vi "Set_Hi-Tec_server.vi"(4 "Client Name":string, 6 "Density Ratio":string, 7 "Strength (% by volume)":dbl min=0.0 max=5.0 format="%.3f", 8 "Stack flowrate (l/min)":dbl format="%.2f", 9 "Mode":enum16{"Control Hi-Tec", "Check Hi-Tec Demands"}(ring)) -> (0 "Flowrates (kg/min)":dbl[](array[numeric]) format="%.2f", 1 "Comment":string)   [LabVIEW 2010]
uses:
  ADAM Client/Sub VIs/ADAM Controls/Update_scan_value.ctl
  ADAM Client/Sub VIs/ADAM Controls/Ch_description_ADAM.ctl
  ADAM Client/Sub VIs/ADAM Controls/Module_type_ADAM.ctl
  ADAM Client/Sub VIs/ADAM Controls/Function_ADAM.ctl
  ADAM Client/Sub VIs/ADAM Controls/Channel_State.ctl
  ADAM Client/Sub VIs/ADAM Controls/Calib_type_ADAM.ctl
  ADAM Client/Sub VIs/ADAM Controls/Address.ctl
  Anemometry/Anemometry Sub Vis/Globals/Gas_management_global.vi
panel:
  # "-Carrier 1 only\n-Carrier 2 only\n-Enter Ratio"
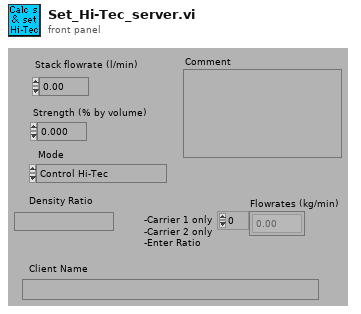
[diagram p1: front panel]
types:
  T1 = enum16{"Append to Global", "Read Global then Clear"}
  T2 = typedef "Ch_description_ADAM.ctl" = cluster{"Ch Name":string, "Type":T3, "Function":T4, "Ch State":T5, "Calibration type":T6, "A":dbl, "B":dbl, "C":dbl, "D":dbl, "Comments":string, "Address":T7, "String":string, "Duty":u16}
  T3 = typedef "Module_type_ADAM.ctl" = enum16{"4011", "4012", "4013", "4014", "4016", "4017", "4018", "4021", "4050", "4052", "4053", "4060", "4080", "5000", "5017", "5018", "5024", "5051", "5056", "5060", "6060", "Tracker", "WEST", "GILL", "JEM", "VICI", "Vaisala", "DRUCK", "Run VI Named:", "IR2100", "PPT", "Comparator", "VIRTUAL", "Hold Value", "Read A", "Read Ch", "Coded", "Client Info", "Web Client", "X10", "Test"}
  T4 = typedef "Function_ADAM.ctl" = enum16{"Analogue Input", "Digital Input", "Event counter", "Event rate", "Analogue Output", "Digital Output", "Relay Output"}
  T5 = typedef "Channel_State.ctl" = enum16{"On", "Off", "Always On", "Always Off"}
  T6 = typedef "Calib_type_ADAM.ctl" = enum16{"Raw", "Bx + A", "Cx^2 + Bx + A", "Dx^3 + Cx^2 + Bx + A", "In Band", "Hi-Tec Q", "Hi-Tec M_dot", "Text"}
  T7 = typedef "Address.ctl" = cluster{"Main":i32, "Ch.":i32, "Sub":i32, "Port Name":string}
  T8 = typedef "Update_scan_value.ctl" = cluster{"Channel Name":string, "New Value":dbl}
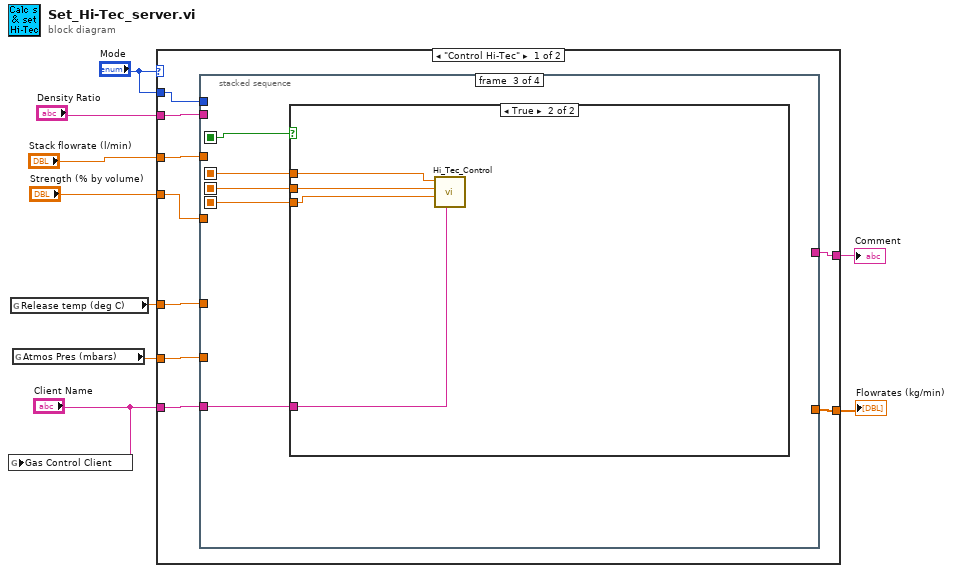
[diagram p0: block diagram]
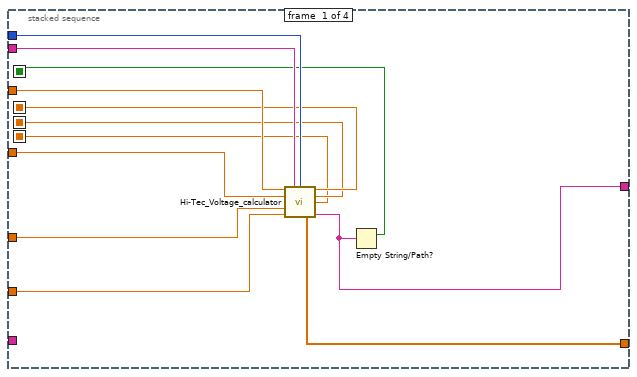
[diagram p2: hidden frame]
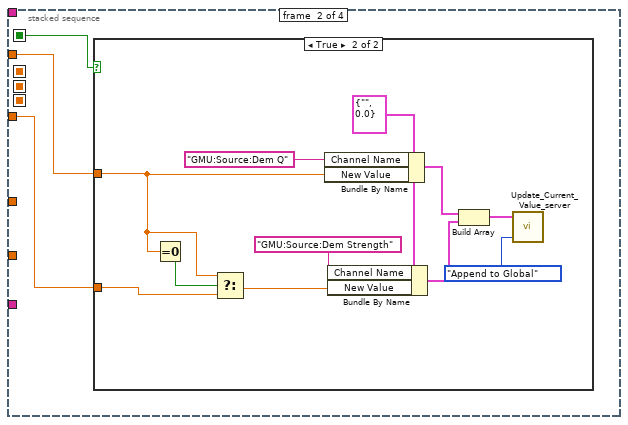
[diagram p3: hidden frame]
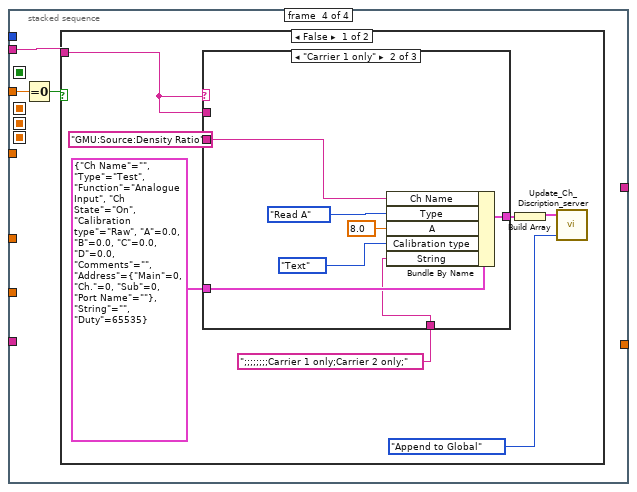
[diagram p6: hidden frame]
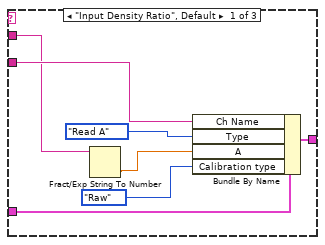
[diagram p7: hidden frame]
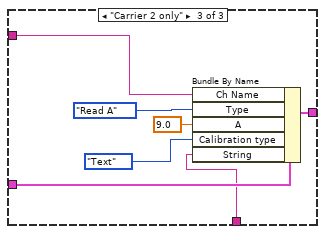
[diagram p8: hidden frame]
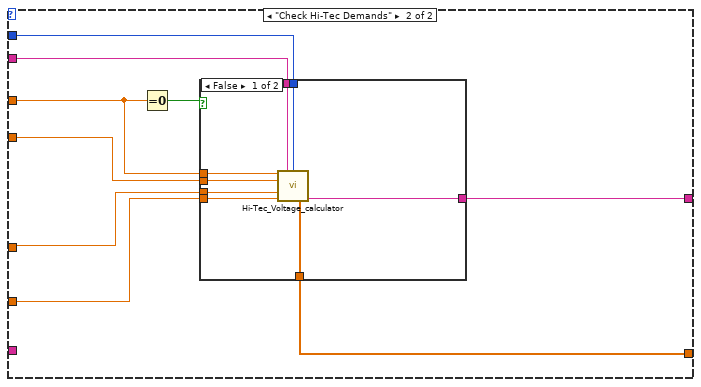
[diagram p10: hidden frame]
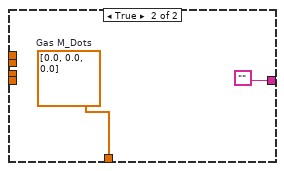
[diagram p11: hidden frame]
diagram:
  n1 = global write "Gas_management_global.vi" "Gas Control Client"("Client Name") -> ()
  n2 = global read "Gas_management_global.vi" "Release temp (deg C)"() -> (w5:dbl)
  n3 = global read "Gas_management_global.vi" "Atmos Pres (mbars)"() -> (w7:dbl)
  n4 = case shown="\"Control Hi-Tec\"" "Mode" {
    tunnel: "Density Ratio" -> [w18 w90]
    tunnel: "Strength (% by volume)" -> [w17 w93]
    tunnel: "Stack flowrate (l/min)" -> [w16 w88]
    tunnel: w5 -> [w15 w92]
    tunnel: w7 -> [w14 w91]
    tunnel: [w13 w89] -> w6
    tunnel: [w12 w86] -> w3
    tunnel: "Mode" -> [w11 w85]
    tunnel: "Client Name" -> [w10 _]
    frame "Control Hi-Tec" {
      n5 = stacked-sequence {
        seq-local: [w22 _ _ _] -> [_ w31 w45 _]
        seq-local: [w21 _ _ _] -> [_ _ w49 _]
        seq-local: [w20 _ _ _] -> [_ _ w48 _]
        seq-local: [w19 _ _ _] -> [_ _ w47 _]
        tunnel: w18 -> [w28 _ _ w56]
        tunnel: w17 -> [w27 w32 _ _]
        tunnel: w16 -> [w26 w33 _ w55]
        tunnel: w15 -> [w30 _ _ _]
        tunnel: w14 -> [w29 _ _ _]
        tunnel: [w23 _ _ _] -> w13
        tunnel: [w25 _ _ _] -> w12
        tunnel: w11 -> [w24 _ _ _]
        tunnel: w10 -> [_ _ w46 _]
        frame #0 {
          n6 = call "Hi-Tec_Voltage_calculator.vi"("Stack Flowrate (l/min)"=w26, "Density Ratio"=w28, "Mode"=w24, "Strength (% by volume)"=w27, "Release temp (deg C)"=w30, "Atmos Pres (mbars)"=w29) -> ("Carrier 1 Voltage"=w21:dbl, "Carrier 2 Voltage"=w20:dbl, "Trace Voltage"=w19:dbl, "Flowrates (kg/min)"=w25:dbl[], "Error Comments"=w23:string)  [unwired: 2 in, 3 out]
          n7 = Empty String/Path?(string/path=w23) -> (empty?=w22:bool)
        }
        frame #1 {
          n8 = case shown="True" w31 {
            tunnel: w33 -> [_ w44]
            tunnel: w32 -> [_ w43]
            frame False {
            }
            frame True {
              w38 = T8 {"Channel Name"="", "New Value"=0.0} ("Update Scan Value Cluster")
              n9 = Equal To 0?(x=w44) -> (x = 0?=w35:bool)
              n10 = Select(t=w44, s=w35, f=w43) -> (s? t:f=w34:dbl)
              n11 = Bundle By Name(cluster=w38, "Channel Name"="GMU:Source:Dem Q", "New Value"=w44) -> (w41:T8)
              n12 = Bundle By Name(cluster=w38, "Channel Name"="GMU:Source:Dem Strength", "New Value"=w34) -> (w42:T8)
              n13 = Build Array(w41, w42) -> (w37:T8[])
              n14 = call "Update_Current_Value_server.vi"("Mode"=T1."Append to Global", "Update array in"=w37) -> ()  [unwired: 1 in, 1 out]
            }
          }
        }
        frame #2 {
          n15 = case shown="True" w45 {
            tunnel: w49 -> [_ w53]
            tunnel: w48 -> [_ w52]
            tunnel: w47 -> [_ w51]
            tunnel: w46 -> [_ w50]
            frame False {
            }
            frame True {
              n16 = call "Hi_Tec_Control.vi"("Carrier 1 Voltage"=w53, "Carrier 2 Voltage"=w52, "Trace Voltage"=w51, "Client Name"=w50) -> ()  [unwired: 3 out]
            }
          }
        }
        frame #3 {
          n17 = Equal To 0?(x=w55) -> (x = 0?=w54:bool)
          n18 = case shown="False" w54 {
            tunnel: w56 -> [w58 _]
            frame False {
              n19 = case shown="\"Carrier 1 only\"" w58 {
                tunnel: T2 {"Ch Name"="", "Type"=enum."Test", "Function"=enum."Analogue Input", "Ch State"=enum."On", "Calibration type"=enum."Raw", "A"=0.0, "B"=0.0, "C"=0.0, "D"=0.0, "Comments"="", "Address"={"Main"=0, "Ch."=0, "Sub"=0, "Port Name"=""}, "String"="", "Duty"=65535} ("Ch Discription") -> [w70 w77 w84]
                tunnel: "GMU:Source:Density Ratio" -> [w69 w76 w83]
                tunnel: [w66 w72 w79] -> w61
                tunnel: w58 -> [w64 _ _]
                tunnel: ";;;;;;;;Carrier 1 only;Carrier 2 only;" -> [_ w71 w78]
                frame "Input Density Ratio", Default {
                  n20 = Fract/Exp String To Number(string=w64) -> (number=w65:dbl)  [unwired: 4 out]
                  n21 = Bundle By Name(cluster=w70, "Ch Name"=w69, "Type"=Module_type_ADAM."Read A", "A"=w65, "Calibration type"=Calib_type_ADAM."Raw") -> (w66:T2)
                }
                frame "Carrier 1 only" {
                  n22 = Bundle By Name(cluster=w77, "Ch Name"=w76, "Type"=Module_type_ADAM."Read A", "A"=8.0 ("Bundle Element"), "Calibration type"=Calib_type_ADAM."Text", "String"=w71) -> (w72:T2)
                }
                frame "Carrier 2 only" {
                  n23 = Bundle By Name(cluster=w84, "Ch Name"=w83, "Type"=Module_type_ADAM."Read A", "A"=9.0 ("Bundle Element"), "Calibration type"=Calib_type_ADAM."Text", "String"=w78) -> (w79:T2)
                }
              }
              n24 = Build Array(w61) -> (w60:T2[])
              n25 = call "Update_Ch_Discription_server.vi"("Mode"=T1."Append to Global", "Channels to update In"=w60) -> ()  [unwired: 1 in, 1 out]
            }
            frame True {
            }
          }
        }
      }
    }
    frame "Check Hi-Tec Demands" {
      n26 = Equal To 0?(x=w88) -> (x = 0?=w87:bool)
      n27 = case shown="False" w87 {
        tunnel: w93 -> [w101 _]
        tunnel: w92 -> [w100 _]
        tunnel: w91 -> [w99 _]
        tunnel: w90 -> [w98 _]
        tunnel: [w97 ""] -> w89
        tunnel: w88 -> [w96 _]
        tunnel: [w95 w102] -> w86
        tunnel: w85 -> [w94 _]
        frame False {
          n28 = call "Hi-Tec_Voltage_calculator.vi"("Stack Flowrate (l/min)"=w96, "Density Ratio"=w98, "Mode"=w94, "Strength (% by volume)"=w101, "Release temp (deg C)"=w100, "Atmos Pres (mbars)"=w99) -> ("Flowrates (kg/min)"=w95:dbl[], "Error Comments"=w97:string)  [unwired: 1 in, 7 out]
        }
        frame True {
          w102 = dbl[] [0.0, 0.0, 0.0]  # Gas M_Dots
        }
      }
    }
  }
  "Comment" <- w6
  "Flowrates (kg/min)" <- w3
